vi "NanotecSMCPD.get addresses.vi"(0 "i ref in":refnum<vi>, 5 "error in (no error)":errorcluster) -> (14 "i ref out":refnum<vi>, 16 "controllerAddresses":i32[](array[numeric]), 19 "error out":errorcluster)   [LabVIEW 2014, in "NanotecSMCPD.lvlib"]
doc: "Gets the addresses of the controllers connected to the interface."
uses:
  NanotecSMCPD.lvlib
  CS_Core/BaseProcess/BaseProcess.lvlib
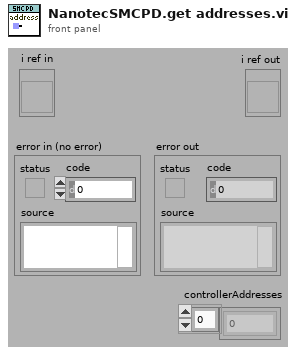
[diagram p1: front panel]
types:
  T1 = typedef "BaseProcess.lvlib/BaseProcess.i attribute.ctl" = cluster{"EventStatus":string, "EventError":i32, "PresetEvtWatchD":i32, "PresetPdcWatchD":i32, "EventTimeout":i32, "PeriodicInterval":i32, "Interface":string[], "Address":string[], "Special":string[], "PeriodicError":i32, "PeriodicStatus":string, "SuperProc":string, "Descriptors":T2[], "CaseRef":refnum<vi>, "PdcRef":refnum<vi>, "Thread Ref":refnum<vi>, "eventErrorID":i32, "eventStatusID":i32, "periodicErrorID":i32, "periodicStatusID":i32, "pdcCtrID":i32}
  T2 = typedef "BaseProcess.lvlib/BaseProcess.descriptor definition.ctl" = cluster{"selector":string, "descriptor":T3}
  T3 = typedef "BaseProcess.lvlib/BaseProcess.descriptor string definition.ctl" = string
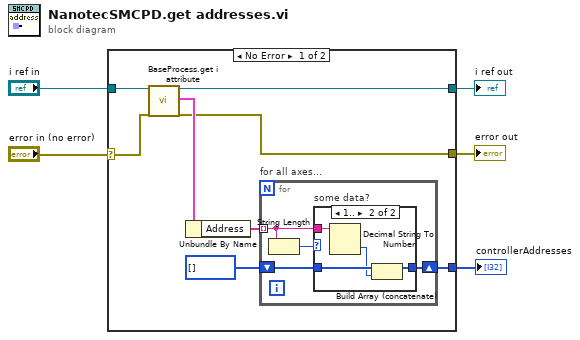
[diagram p0: block diagram]
diagram:
  n1 = case shown="No Error" "error in (no error)" {
    selector: "error in (no error)" -> [w9 w23]
    tunnel: "i ref in" -> [w13 w24]
    tunnel: [w11 w24] -> w4
    tunnel: [w10 w23] -> w3
    tunnel: [w6 _] -> w2
    frame No Error {
      n2 = call "BaseProcess.get i attribute.vi"("i ref in"=w13, "error in (no error)"=w9) -> ("i ref out"=w11:refnum<vi>, "i attribute"=w12:T1, "error out"=w10:errorcluster)  [unwired: 15 in]
      n3 = Unbundle By Name(w12) -> ("Address"=w8:string[])
      n4 = for "for all axes..." {
        tunnel: w8 -> [w17] mode=indexing
        shift-right: [w14] -> w6
        shift-left: i32[] [] -> [w15]
        n5 = String Length(string=w17) -> (length=w16:i32)
        n6 = case "some data?" shown="1.." w16 {
          tunnel: w17 -> [_ w22]
          tunnel: w15 -> [w18 w21]
          tunnel: [w18 w19] -> w14
          frame 0, Default {
          }
          frame 1.. {
            n7 = Decimal String To Number(string=w22) -> (number=w20:i32)  [unwired: 2 in, 1 out]
            n8 = Build Array (concatenate)(w21, w20) -> (w19:i32[])
          }
        }
      }
    }
    frame Error {
    }
  }
  "error out" <- w3
  "i ref out" <- w4
  "controllerAddresses" <- w2
